vi "Send.vi"(10 "Panel":refnum<class "Panel.lvclass">) -> (3 "Panel Create Msg out":refnum<class "Panel Create Msg.lvclass">)   [LabVIEW 2021, in "Panel Create.lvlib" / "Panel Create Msg.lvclass"]
uses:
  Panel Create Msg.lvclass
  Panel/Panel.lvclass
  Panel Create Msg.lvclass/Panel Create Msg.ctl
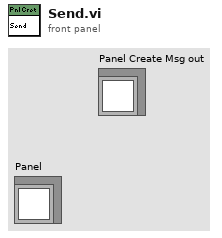
[diagram p1: front panel]
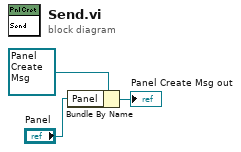
[diagram p0: block diagram]
diagram:
  n1 = Bundle By Name(cluster=refnum<class "Panel Create Msg.lvclass"> refnum ("Panel Create Msg Strategy out"), "Panel"="Panel") -> (→"Panel Create Msg out":refnum<class "Panel Create Msg.lvclass">)
